vi "CreateReportFiles.vi"(8 "error in":errorcluster) -> (0 "error out":errorcluster)   [LabVIEW 2018, in "S2.lvclass"]
uses:
  S2.lvclass
  Queue/Queue Data.ctl
  Queue/State.ctl
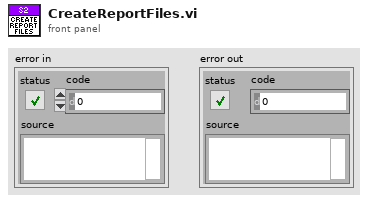
[diagram p1: front panel]
types:
  T1 = typedef "S2.lvclass/Queue Data.ctl" = cluster{"State":T2, "Data":variant}
  T2 = typedef "S2.lvclass/State.ctl" = enum16{"Initialize", "SetConfig", "AckAlarm", "Alarm", "Idle", "LockLid", "LowPressure", "Pressurize", "DecayTest", "Vent", "Abort", "Start", "CreateReports", "WriteToReport", "WritePressure", "Error", "Exit"}
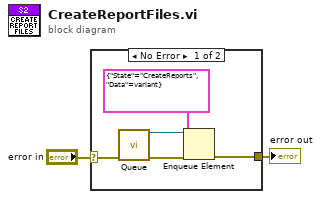
[diagram p0: block diagram]
diagram:
  n1 = case shown="No Error" "error in" {
    selector: "error in" -> [w7 w8]
    tunnel: [w4 w8] -> w2
    frame No Error {
      n2 = call "Queue.vi"("error in"=w7) -> ("error out"=w6:errorcluster, "queue out"=w5:refnum<queue>)  [unwired: 9 in]
      n3 = Enqueue Element(queue=w5, element=T1 {"State"=enum."CreateReports", "Data"=variant}, error in (no error)=w6) -> (error out=w4:errorcluster)  [unwired: 1 in, 2 out]
    }
    frame Error {
    }
  }
  "error out" <- w2
